vi "Calculator.vi"() -> ()   [LabVIEW 2018]
uses:
  <vilib>/gmath/SpecialFunctions.llb/Gamma Function.vi
  <vilib>/regexp/Match Regular Expression.xnode
  <vilib>/gmath/NI_Gmath.lvlib
panel:
  in  "Boton .":bool
  in  "Boton nqrt":bool
  in  "Boton sqrt":bool
  in  "Boton e":bool
  in  "boton asen":bool
  in  "Boton crt":bool
  in  "Boton tan(x)":bool
  in  "Boton cos(x)":bool
  in  "Boton sen(x)":bool caption="1"
  in  "Boton tanh":bool
  in  "Boton cosh":bool
  in  "Boton sech":bool caption="1"
  in  "Boton Pi":bool
  in  "Boton atan":bool
  in  "Boton acos":bool
  in  "Boton R2D":bool
  in  "Boton D2R":bool
  in  "Boton Log(x)":bool
  in  "Boton Ln":bool
  in  "Boton Log":bool caption="1"
  in  "Boton x^y":bool
  in  "Boton x^3":bool
  in  "Boton x^2":bool caption="1"
  in  "Boton x^-1":bool
  in  "Boton e^x":bool
  in  "Boton x!":bool caption="1"
  in  "Boton )":bool
  in  "Boton (":bool
  in  "Boton /":bool
  in  "Boton *":bool
  in  "Boton -":bool
  in  "Boton =":bool
  in  "Boton +":bool
  in  "Boton Ans":bool
  out "Pantalla":string
  in  "Boton 0":bool
  in  "Boton DEL":bool
  in  "Boton C":bool
  in  "Boton 9":bool
  in  "Boton 8":bool
  in  "Boton 7":bool
  in  "Boton 6":bool
  in  "Boton 5":bool
  in  "Boton 4":bool
  in  "Boton 3":bool
  in  "Boton 2":bool
  in  "Boton 1":bool caption="1"
  out "Boolean":bool
  out "Del":bool
  out "result string":string
  in  "Ans":dbl
  # "CALCULATOR \nDIEGO ALEJANDRO HENAO JIMENEZ\nHUGO ANDRES TORRES\nPOLITECNICO JAIME IZASA CADAVID"
  # "La Funcion LOG , es la que evalua logaritmos en base n, Para su implementacion se sugiere ingresarla\nde esta manera LOG20(0,1), Se sugiere que cerrar debidamente las funciones con parentesis."
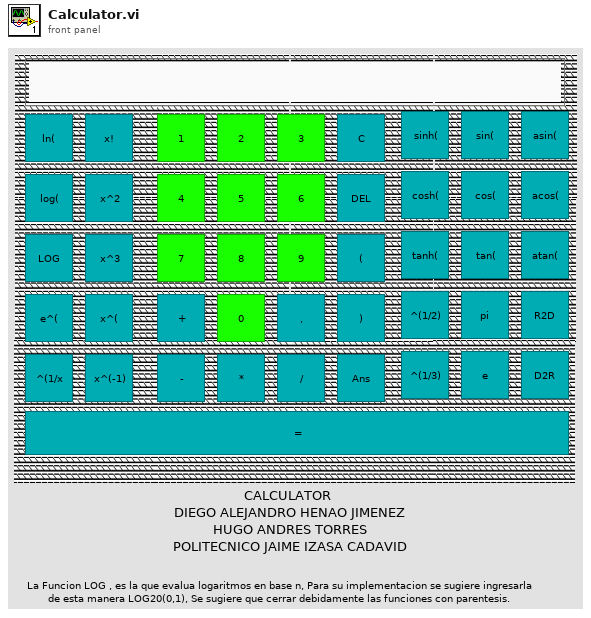
[diagram p1: front panel]
types:
  T1 = typedef "eventvkey.ctl" = enum16{"ASCII", "Enter", "Return", "Shift", "Ctrl", "Alt", "Cmd", "Opt", "Caps", "NumLock", "Clear", "Break", "Up", "Down", "Left", "Right", "Insert", "Delete", "Home", "End", "PageUp", "PageDown", "Escape", "Help", "Pause", "ScrollLock", "F1", "F2", "F3", "F4", "F5", "F6", "F7", "F8", "F9", "F10", "F11", "F12", "F13", "F14", "F15", "F16", "F17", "F18", "F19", "F20", "F21", "F22", "F23", "F24", "Play", "VolumeUp", "VolumeDown", "Mute", "Two Byte Char"}
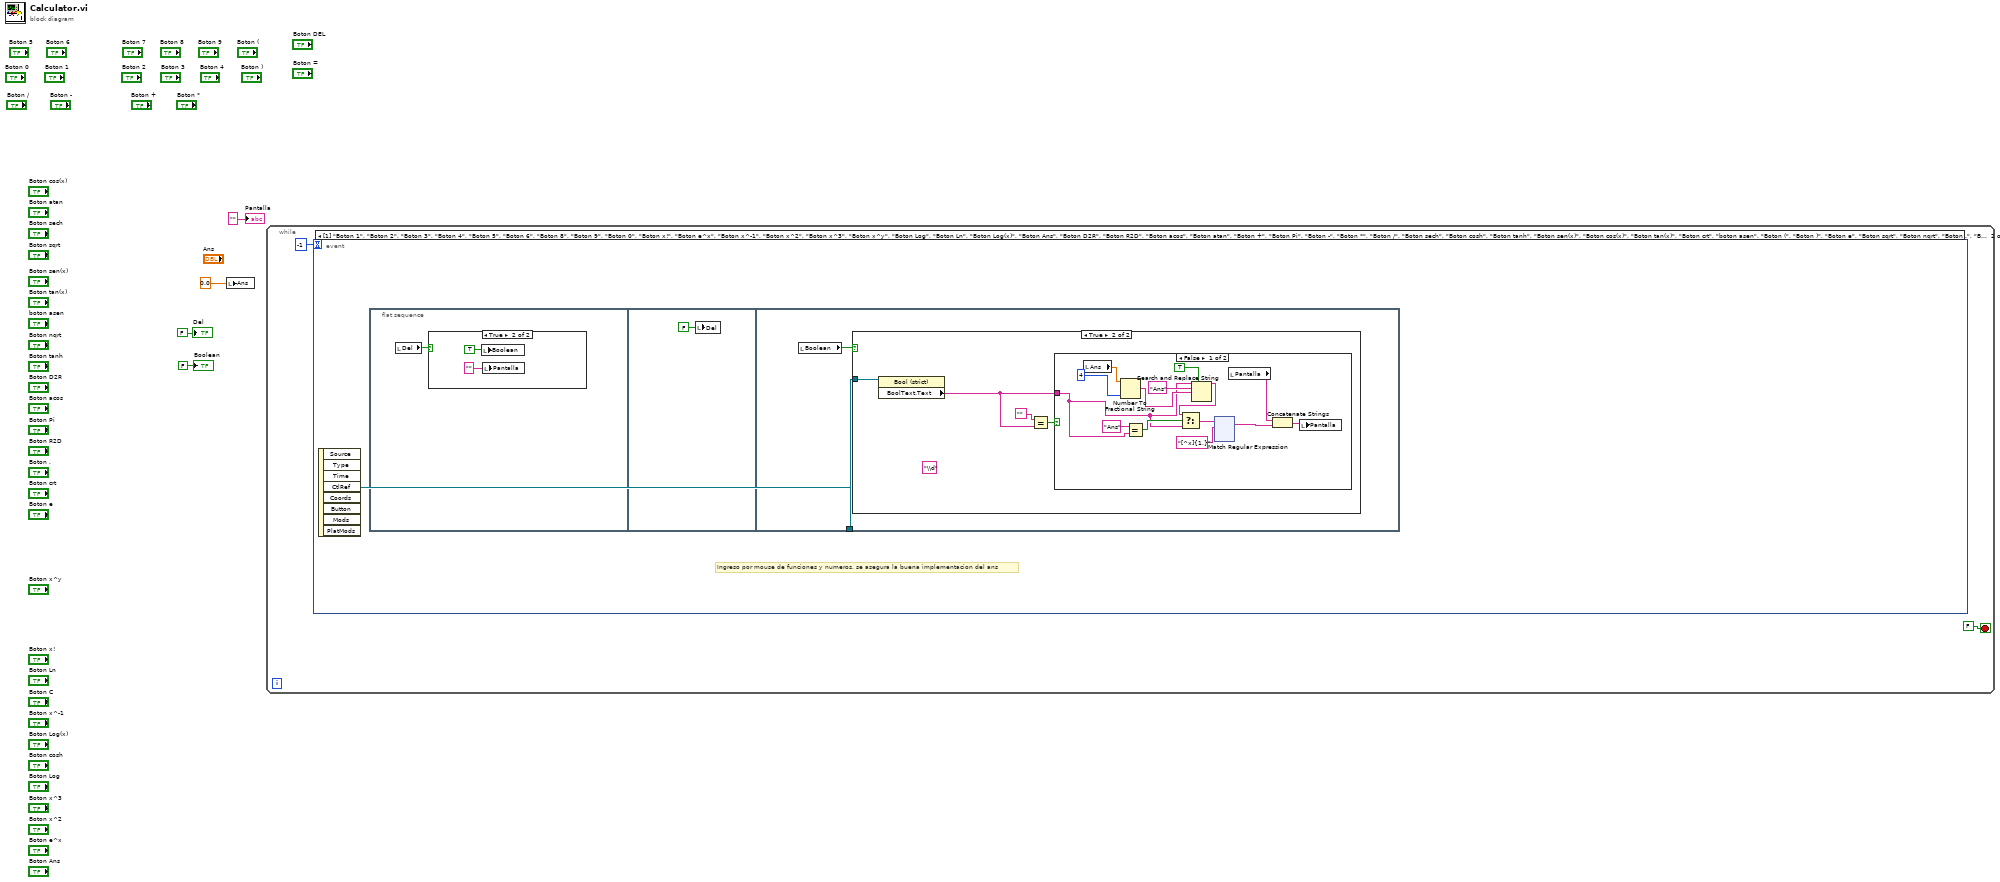
[diagram p0: block diagram]
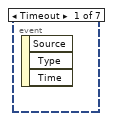
[diagram p2: hidden frame]
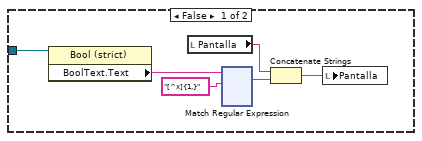
[diagram p4: hidden frame]
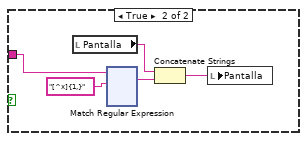
[diagram p5: hidden frame]
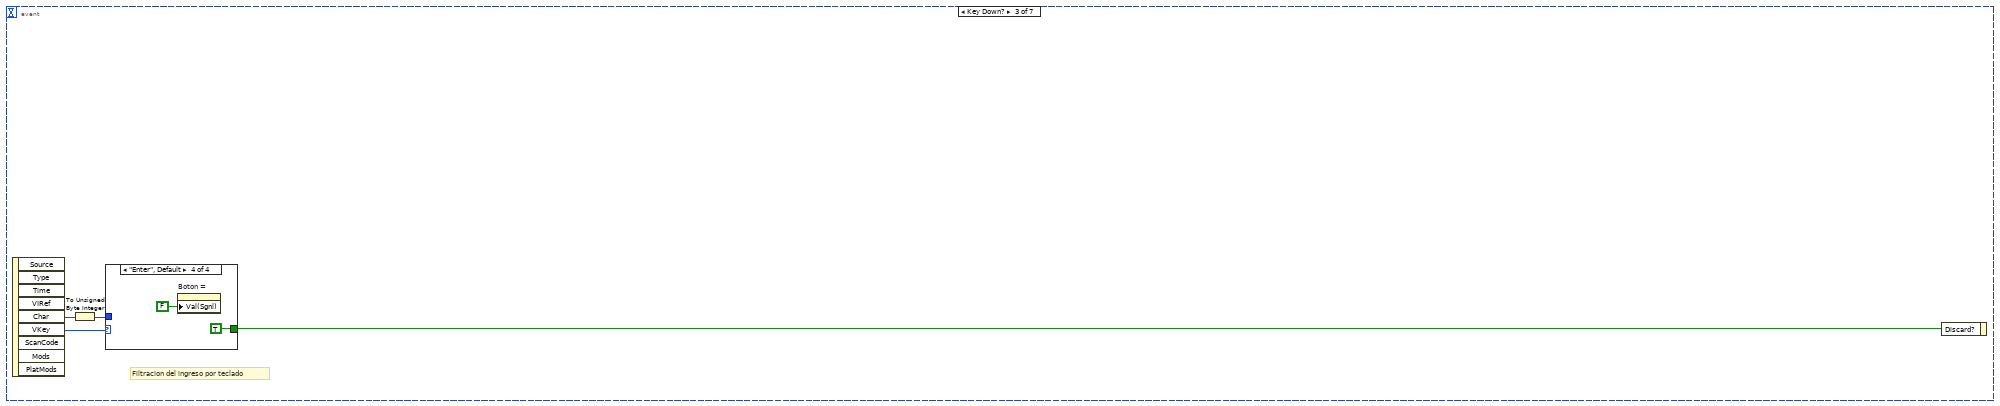
[diagram p6: hidden frame]
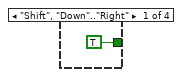
[diagram p7: hidden frame]
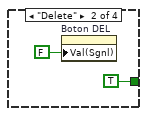
[diagram p8: hidden frame]
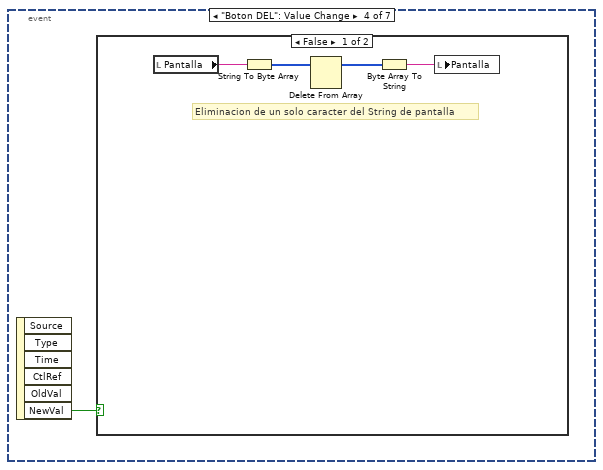
[diagram p10: hidden frame]
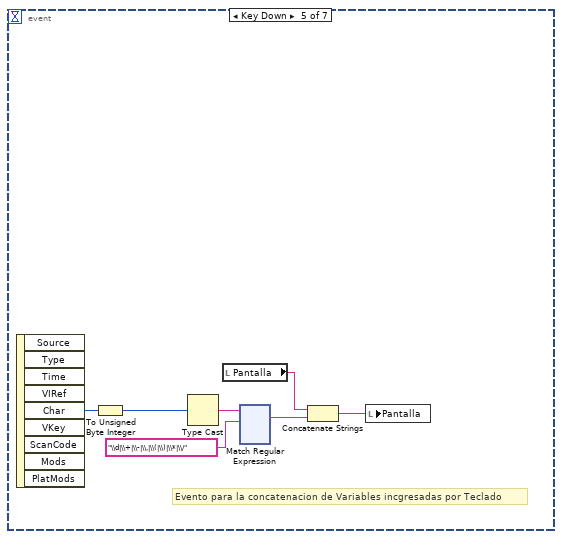
[diagram p12: hidden frame]
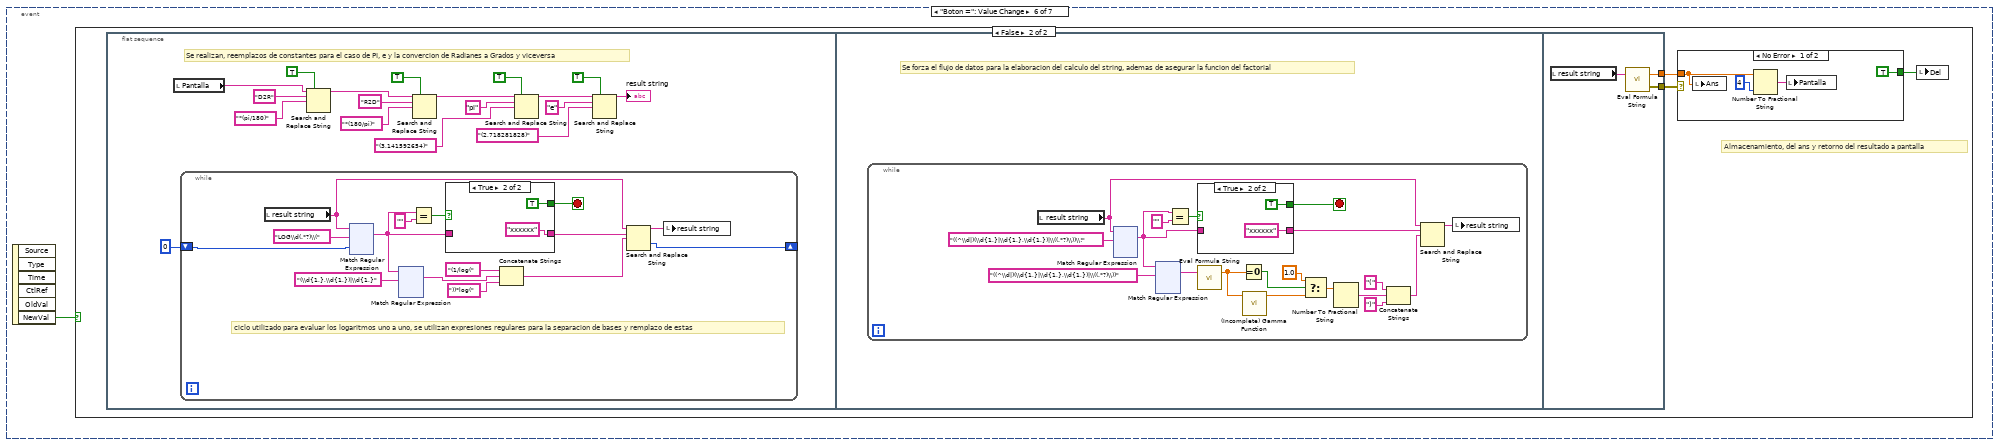
[diagram p13: hidden frame]
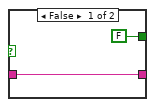
[diagram p15: hidden frame]
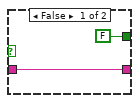
[diagram p16: hidden frame]
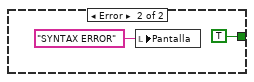
[diagram p17: hidden frame]
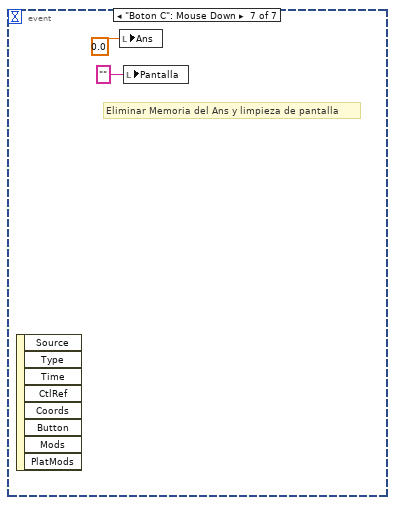
[diagram p18: hidden frame]
diagram:
  n1 = local write "Ans"(0.0) -> ()
  n2 = while {
    stop <- FALSE stop-if-true
    n3 = event shown="[1] \"Boton 1\", \"Boton 2\", \"Boton 3\", \"Boton 4\", \"Boton 5\", \"Boton 6\", \"Boton 8\", \"Boton 9\", \"Boton 0\", \"Boton x!\", \"Boton e^x\", \"Boton x^-1\", \"Boton x^2\", \"Boton x^3\", \"Boton x^y\", \"Boton Log\", \"Boton Ln\", \"Boton Log(x)\", \"Boton Ans\", \"Boton D2R\", \"Boton R2D\", \"Boton acos\", \"Boton atan\", \"Boton +\", \"Boton Pi\", \"Boton -\", \"Boton *\", \"Boton /\", \"Boton sech\", \"Boton cosh\", \"Boton tanh\", \"Boton sen(x)\", \"Boton cos(x)\", \"Boton tan(x)\", \"Boton crt\", \"boton asen\", \"Boton (\", \"Boton )\", \"Boton e\", \"Boton sqrt\", \"Boton nqrt\", \"Boton .\", \"Boton 7\": Mouse Down" {
      selector: _ -> [_ _ _ _ _ _ _]
      dyn-events: _ -> [_ _ _ _ _ _ _]
      timeout: -1 -> [_ _ _ _ _ _ _]
      event Timeout {
        n4 = event-data() -> ()  [unwired: 1 in, 3 out]
      }
      event "Boton 1", "Boton 2", "Boton 3", "Boton 4", "Boton 5", "Boton 6", "Boton 8", "Boton 9", "Boton 0", "Boton x!", "Boton e^x", "Boton x^-1", "Boton x^2", "Boton x^3", "Boton x^y", "Boton Log", "Boton Ln", "Boton Log(x)", "Boton Ans", "Boton D2R", "Boton R2D", "Boton acos", "Boton atan", "Boton +", "Boton Pi", "Boton -", "Boton *", "Boton /", "Boton sech", "Boton cosh", "Boton tanh", "Boton sen(x)", "Boton cos(x)", "Boton tan(x)", "Boton crt", "boton asen", "Boton (", "Boton )", "Boton e", "Boton sqrt", "Boton nqrt", "Boton .", "Boton 7": Mouse Down {
        # "Ingreso por mouse de funciones y numeros, se asegura la buena implementacion del ans"
        n5 = event-data() -> ("CtlRef"=w7:refnum<vi>)  [unwired: 1 in, 7 out]
        n6 = flat-sequence {
          tunnel: w7 -> [w12]
          frame #0 {
            n7 = local read "Del"() -> (w8:bool)
            n8 = case shown="True" w8 {
              frame False {
              }
              frame True {
                n9 = local write "Boolean"(TRUE ("Boolean")) -> ()
                n10 = local write "Pantalla"("" ("Pantalla")) -> ()
              }
            }
          }
          frame #1 {
            n11 = local write "Del"(FALSE ("Del")) -> ()
          }
          frame #2 {
            n12 = local read "Boolean"() -> (w13:bool)
            n13 = case shown="True" w13 {
              tunnel: w12 -> [w14 w137]
              frame False {
                n14 = property class="Bool (strict)"(reference=w14) -> ("BoolText.Text"=w18:string)  [unwired: 1 in, 2 out]
                n15 = local read "Pantalla"() -> (w19:string)
                n16 = xnode "Match Regular Expression"("input string"=w18, "regular expression"="[^x]{1,}") -> ("whole match"=w17:string)  [unwired: 4 in, 4 out]
                n17 = Concatenate Strings(w19, w17) -> (w16:string)
                n18 = local write "Pantalla"(w16) -> ()
              }
              frame True {
                (unwired) "\\d" ("regular expression")
                n19 = property class="Bool (strict)"(reference=w137) -> ("BoolText.Text"=w134:string)  [unwired: 1 in, 2 out]
                n20 = Equal?(x="", y=w134) -> (x = y?=w135:bool)
                n21 = case shown="False" w135 {
                  tunnel: w134 -> [w138 w266]
                  frame False {
                    n22 = local read "Ans"() -> (w143:dbl)
                    n23 = Number To Fractional String(number=w143, precision (6)=i16 4) -> (F-format string=w140:string)  [unwired: 2 in]
                    n24 = Equal?(x="Ans", y=w138) -> (x = y?=w146:bool)
                    n25 = Search and Replace String(replace all?=TRUE ("replace all? (F)"), input string=w138, search string="Ans", replace string=w140) -> (result string=w139:string)  [unwired: 4 in, 3 out]
                    n26 = Select(t=w139, s=w146, f=w138) -> (s? t:f=w144:string)
                    n27 = xnode "Match Regular Expression"("input string"=w144, "regular expression"="[^x]{1,}") -> ("whole match"=w150:string)  [unwired: 4 in, 4 out]
                    n28 = local read "Pantalla"() -> (w148:string)
                    n29 = Concatenate Strings(w148, w150) -> (w151:string)
                    n30 = local write "Pantalla"(w151) -> ()
                  }
                  frame True {
                    n31 = local read "Pantalla"() -> (w270:string)
                    n32 = xnode "Match Regular Expression"("input string"=w266, "regular expression"="[^x]{1,}") -> ("whole match"=w269:string)  [unwired: 4 in, 4 out]
                    n33 = Concatenate Strings(w270, w269) -> (w268:string)
                    n34 = local write "Pantalla"(w268) -> ()
                  }
                }
              }
            }
          }
        }
      }
      event Key Down? {
        # "Filtracion del ingreso por teclado"
        n35 = event-data() -> ("Char"=w388:i16, "VKey"=w387:T1)  [unwired: 1 in, 7 out]
        n36 = To Unsigned Byte Integer(number=w388) -> (unsigned 8bit integer=w386:u8)
        n37 = case shown="\"Enter\", Default" w387 {
          tunnel: w386 -> [_ _ _ _]
          tunnel: [TRUE ("Value (Signaling)") TRUE ("Value (Signaling)") _ TRUE ("Value (Signaling)")] -> w385
          frame "Shift", "Down".."Right" {
          }
          frame "Delete" {
            n38 = property on="Boton DEL" class="Bool (strict)"("Val(Sgnl)"=FALSE ("Value (Signaling)")) -> ()  [unwired: 2 in, 2 out]
          }
          frame "ASCII" {
          }
          frame "Enter", Default {
            n39 = property on="Boton =" class="Bool (strict)"("Val(Sgnl)"=FALSE ("Value (Signaling)")) -> ()  [unwired: 2 in, 2 out]
          }
        }
        n40 = event-data("Discard?"=w385) -> ()  [unwired: 1 in, 1 out]
      }
      event "Boton DEL": Value Change {
        n41 = event-data() -> ("NewVal"=w394:bool)  [unwired: 1 in, 5 out]
        n42 = case shown="False" w394 {
          frame False {
            # "Eliminacion de un solo caracter del String de pantalla"
            n43 = local read "Pantalla"() -> (w397:string)
            n44 = String To Byte Array(string=w397) -> (unsigned byte array=w398:u8[])
            n45 = Delete From Array(array=w398) -> (array with subset deleted=w396:u8[])  [unwired: 2 in, 1 out]
            n46 = Byte Array To String(unsigned byte array=w396) -> (string=w395:string)
            n47 = local write "Pantalla"(w395) -> ()
          }
          frame True {
          }
        }
      }
      event Key Down {
        # "Evento para la concatenacion de Variables incgresadas por Teclado"
        n48 = event-data() -> ("Char"=w402:i16)  [unwired: 1 in, 8 out]
        n49 = To Unsigned Byte Integer(number=w402) -> (unsigned 8bit integer=w403:u8)
        n50 = Type Cast(x=w403) -> (*(type *) &x=w399:string)  [unwired: 1 in]
        n51 = local read "Pantalla"() -> (w404:string)
        n52 = xnode "Match Regular Expression"("input string"=w399, "regular expression"="\\d|\\+|\\-|\\,|\\(|\\)|\\*|\\/") -> ("whole match"=w400:string)  [unwired: 4 in, 4 out]
        n53 = Concatenate Strings(w404, w400) -> (w405:string)
        n54 = local write "Pantalla"(w405) -> ()
      }
      event "Boton =": Value Change {
        n55 = event-data() -> ("NewVal"=w520:bool)  [unwired: 1 in, 5 out]
        n56 = case shown="False" w520 {
          frame True {
          }
          frame False {
            # "Almacenamiento, del ans y retorno del resultado a pantalla"
            n57 = flat-sequence {
              tunnel: [w1042] -> w523
              tunnel: [w1041] -> w522
              frame #0 {
                # "Se realizan, reemplazos de constantes para el caso de PI, e y la convercion de Radianes a Grados y viceversa"
                n58 = local read "Pantalla"() -> (w527:string)
                n59 = while {
                  shift-right: [w551] -> _
                  shift-left: 0 ("offset past match") -> [w550]
                  stop <- w547 stop-if-true
                  # "ciclo utilizado para evaluar los logaritmos uno a uno, se utilizan expresiones regulares para la separacion de bases y remplazo de estas"
                  n60 = local read "result string"() -> (w545:string)
                  n61 = xnode "Match Regular Expression"("input string"=w545, "regular expression"="LOG\\d(.*?)\\(", "offset (0)"=w550) -> ("whole match"=w544:string)  [unwired: 3 in, 4 out]
                  n62 = xnode "Match Regular Expression"("input string"=w544, "regular expression"="(\\d{1,},\\d{1,})|\\d{1,}") -> ("whole match"=w553:string)  [unwired: 4 in, 4 out]
                  n63 = Equal?(x=w544, y="") -> (x = y?=w549:bool)
                  n64 = case shown="True" w549 {
                    tunnel: [FALSE TRUE] -> w547
                    tunnel: w544 -> [w786 _]
                    tunnel: [w786 "xxxxxx" ("before match")] -> w546
                    frame False {
                    }
                    frame True {
                    }
                  }
                  n65 = Concatenate Strings("(1/log(" ("string"), w553, "))*log(" ("string")) -> (w543:string)
                  n66 = Search and Replace String(input string=w545, search string=w546, replace string=w543) -> (result string=w552:string, offset past replacement=w551:i32)  [unwired: 5 in, 2 out]
                  n67 = local write "result string"(w552) -> ()
                }
                n68 = Search and Replace String(replace all?=TRUE ("replace all? (F)"), input string=w527, search string="D2R", replace string="*(pi/180)" ("replace string (\"\")")) -> (result string=w528:string)  [unwired: 4 in, 3 out]
                n69 = Search and Replace String(replace all?=TRUE ("replace all? (F)"), input string=w528, search string="R2D", replace string="*(180/pi)" ("replace string (\"\")")) -> (result string=w526:string)  [unwired: 4 in, 3 out]
                n70 = Search and Replace String(replace all?=TRUE ("replace all? (F)"), input string=w526, search string="pi", replace string="(3,141592654)" ("replace string (\"\")")) -> (result string=w541:string)  [unwired: 4 in, 3 out]
                n71 = Search and Replace String(replace all?=TRUE ("replace all? (F)"), input string=w541, search string="e", replace string="(2,718281828)" ("replace string (\"\")")) -> (result string=→"result string":string)  [unwired: 4 in, 3 out]
              }
              frame #1 {
                # "Se forza el flujo de datos para la elaboracion del calculo del string, ademas de asegurar la funcion del factorial"
                n72 = while {
                  stop <- w801 stop-if-true
                  n73 = local read "result string"() -> (w807:string)
                  n74 = xnode "Match Regular Expression"("input string"=w807, "regular expression"="((^\\d|)(\\d{1,}|\\d{1,},\\d{1,})|\\((.*?)\\))\\!") -> ("whole match"=w800:string)  [unwired: 4 in, 4 out]
                  n75 = xnode "Match Regular Expression"("input string"=w800, "regular expression"="((^\\d|)(\\d{1,}|\\d{1,},\\d{1,})|\\((.*?)\\))") -> ("whole match"=w806:string)  [unwired: 4 in, 4 out]
                  n76 = Equal?(x=w800, y="") -> (x = y?=w802:bool)
                  n77 = case shown="True" w802 {
                    tunnel: [FALSE TRUE] -> w801
                    tunnel: w800 -> [w809 _]
                    tunnel: [w809 "xxxxxx" ("before match")] -> w799
                    frame False {
                    }
                    frame True {
                    }
                  }
                  n78 = call <vilib>:"Eval Formula String.vi"("formula"=w806) -> ("y value"=w793:dbl)  [unwired: 1 in, 1 out]
                  n79 = Equal To 0?(x=w793) -> (x = 0?=w792:bool)
                  n80 = call-poly <vilib>:"(Incomplete) Gamma Function.vi"("x"=w793) -> ("g(x)"=w790:dbl)  [unwired: 10 in]
                  n81 = Select(t=1.0, s=w792, f=w790) -> (s? t:f=w789:dbl)
                  n82 = Number To Fractional String(number=w789) -> (F-format string=w797:string)  [unwired: 3 in]
                  n83 = Concatenate Strings("(" ("string"), w797, ")" ("string")) -> (w796:string)
                  n84 = Search and Replace String(input string=w807, search string=w799, replace string=w796) -> (result string=w798:string)  [unwired: 5 in, 3 out]
                  n85 = local write "result string"(w798) -> ()
                }
              }
              frame #2 {
                n86 = local read "result string"() -> (w1040:string)
                n87 = call <vilib>:"Eval Formula String.vi"("formula"=w1040) -> ("error out"=w1042:errorcluster, "y value"=w1041:dbl)  [unwired: 1 in]
              }
            }
            n88 = case shown="No Error" w523 {
              tunnel: w522 -> [w1045 _]
              tunnel: [TRUE TRUE] -> w521
              frame No Error {
                n89 = local write "Ans"(w1045) -> ()
                n90 = Number To Fractional String(number=w1045, precision (6)=i16 4) -> (F-format string=w1046:string)  [unwired: 2 in]
                n91 = local write "Pantalla"(w1046) -> ()
              }
              frame Error {
                n92 = local write "Pantalla"("SYNTAX ERROR" ("String")) -> ()
              }
            }
            n93 = local write "Del"(w521) -> ()
          }
        }
      }
      event "Boton C": Mouse Down {
        # "Eliminar Memoria del Ans y limpieza de pantalla"
        n94 = event-data() -> ()  [unwired: 1 in, 8 out]
        n95 = local write "Ans"(0.0 ("Ans")) -> ()
        n96 = local write "Pantalla"("" ("Pantalla")) -> ()
      }
    }
  }
  "Pantalla" <- "" ("String")
  "Del" <- FALSE ("Del")
  "Boolean" <- FALSE ("Boolean")
